vi "tcp_move_abs.vi"(6 "wait4motiondone":bool, 8 "error in (no error)":errorcluster, 9 "destination nm/u°":dbl, 10 "Axis":string(combo), 11 "IP address":string="172.16.6.101") -> (0 "error out":errorcluster, 2 "position":dbl, 3 "IP address out":string="172.16.6.101")   [LabVIEW 2017]
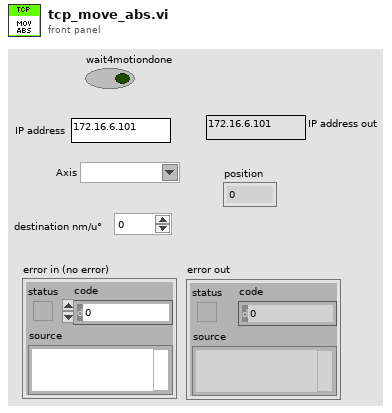
[diagram p1: front panel]
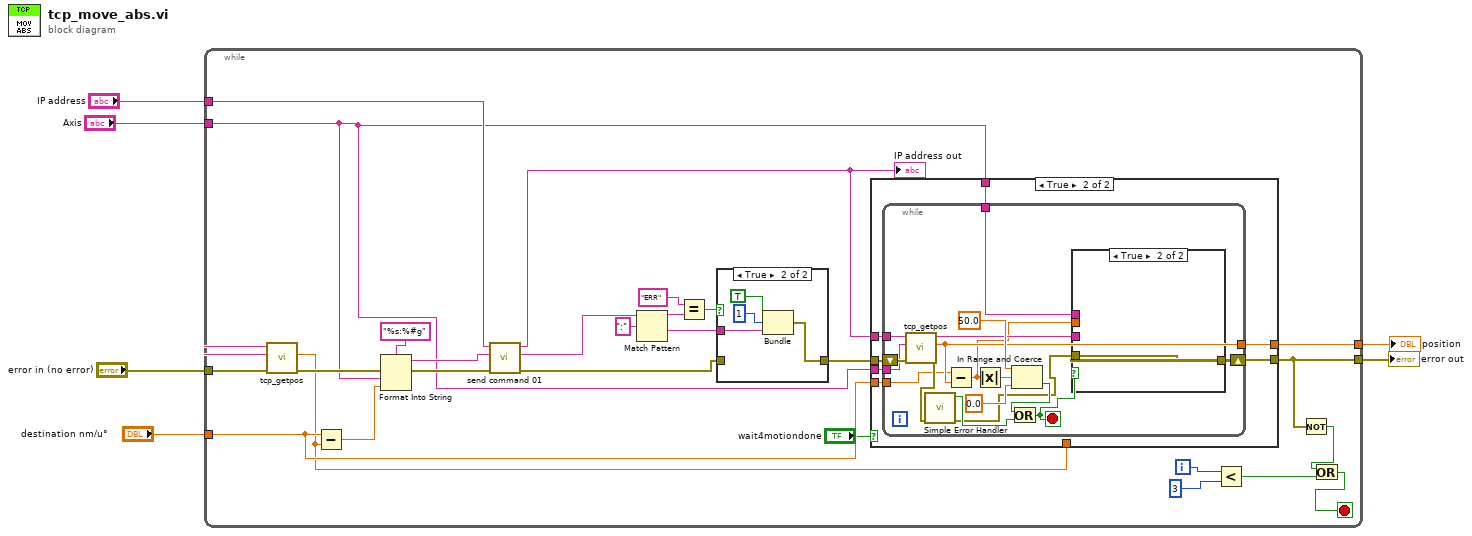
[diagram p0: block diagram]
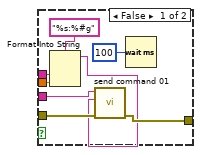
[diagram p3: hidden frame]
diagram:
  n1 = while {
    tunnel: "IP address" -> [w25]
    tunnel: "error in (no error)" -> [w24]
    tunnel: "destination nm/u°" -> [w20]
    tunnel: [w8] -> w3
    tunnel: [w16] -> w2
    tunnel: "Axis" -> [w13]
    i -> [w12]
    stop <- w9 stop-if-true
    n2 = call "tcp_getpos.vi"("error in (no error)"=w24, "Axis"=w13, "IP address"=w25) -> ("error out"=w23:errorcluster, "position"=w17:dbl)  [unwired: 6 in, 1 out]
    n3 = Subtract(x=w20, y=w17) -> (x-y=w15:dbl)
    n4 = Format Into String(format string="%s:%#g", error in=w23, w13, w15) -> (resulting string=w14:string, error out=w22:errorcluster)  [unwired: 1 in]
    n5 = call "send command 01.vi"("error in (no error)"=w22, "command"=w14, "IP address in"=w25) -> ("error out"=w26:errorcluster, "response"=w29:string, "IP address out"=w19:string)  [unwired: 6 in]
    "IP address out" <- w19
    n6 = Match Pattern(string=w29, regular expression=":") -> (before substring=w31:string, after substring=w27:string)  [unwired: 1 in, 2 out]
    n7 = Equal?(x="ERR", y=w31) -> (x = y?=w28:bool)
    n8 = case shown="True" w28 {
      tunnel: w27 -> [_ w71]
      tunnel: [w69 w70] -> w21
      tunnel: w26 -> [w69 _]
      frame False {
      }
      frame True {
        n9 = Bundle(TRUE, 1, "response"=w71) -> (w70:cluster{bool, i32, "response":string})  [unwired: 1 in]
      }
    }
    n10 = case shown="True" "wait4motiondone" {
      tunnel: w21 -> [w35 w42]
      tunnel: w20 -> [_ w41]
      tunnel: w19 -> [_ w40]
      tunnel: w13 -> [_ w39]
      tunnel: [w35 w38] -> w8
      tunnel: [w34 w37] -> w16
      tunnel: w17 -> [w34 _]
      tunnel: w13 -> [_ w36]
      frame False {
      }
      frame True {
        n11 = while {
          tunnel: w40 -> [w59]
          tunnel: w39 -> [w57]
          tunnel: w41 -> [w45]
          shift-right: [w49] -> w38
          shift-left: w42 -> [w58]
          tunnel: [w46] -> w37
          tunnel: w36 -> [w44]
          stop <- w47 stop-if-true
          n12 = call "tcp_getpos.vi"("error in (no error)"=w58, "Axis"=w57, "IP address"=w59) -> ("error out"=w52:errorcluster, "position"=w46:dbl, "IP address out"=w48:string)  [unwired: 6 in]
          n13 = call <vilib>:"Simple Error Handler.vi"("error in (no error)"=w52) -> ("error?"=w51:bool, "error out"=w50:errorcluster)  [unwired: 4 in, 3 out]
          n14 = Subtract(x=w45, y=w46) -> (x-y=w43:dbl)
          n15 = Absolute Value(x=w43) -> (abs(x)=w56:dbl)
          n16 = In Range and Coerce(upper limit=50.0, x=w56, lower limit=0.0) -> (In Range?=w53:bool)  [unwired: 1 out]
          n17 = Or(x=w53, y=w51) -> (x .or. y?=w47:bool)
          n18 = case shown="True" w47 {
            tunnel: w50 -> [w67 w68]
            tunnel: [w66 w68] -> w49
            tunnel: w48 -> [w65 _]
            tunnel: w44 -> [w62 _]
            tunnel: w43 -> [w61 _]
            frame False {
              n19 = Format Into String(format string="%s:%#g", w62, w61) -> (resulting string=w60:string)  [unwired: 2 in, 1 out]
              n20 = call "send command 01.vi"("error in (no error)"=w67, "command"=w60, "IP address in"=w65) -> ("error out"=w66:errorcluster)  [unwired: 6 in, 2 out]
              n21 = Wait (ms)(milliseconds to wait=u32 100) -> ()  [unwired: 1 out]
            }
            frame True {
            }
          }
        }
      }
    }
    n22 = Less?(x=w12, y=3) -> (x < y?=w10:bool)
    n23 = Not(x=w8) -> (.not. x?=w7:bool)
    n24 = Or(x=w7, y=w10) -> (x .or. y?=w9:bool)
  }
  "error out" <- w3
  "position" <- w2
